vi "Get value by Variant.vi"(8 "error in (no error)":errorcluster, 11 "By-Value Column in":refnum<class "By-Value Column.lvclass">) -> (0 "error out":errorcluster, 2 "Variant":variant, 3 "By-Value Column out":refnum<class "By-Value Column.lvclass">)   [LabVIEW 2020, in "Basic Columns.lvlib" / "By-Value Column.lvclass"]
uses:
  By-Value Column.lvclass
  Column Class/Column Parent.lvclass
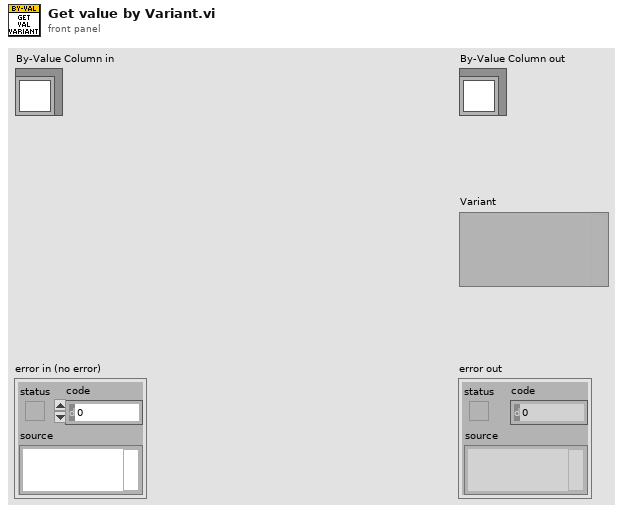
[diagram p1: front panel]
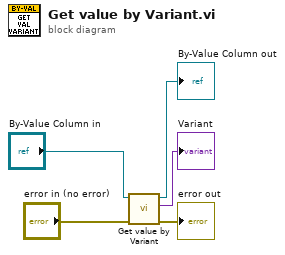
[diagram p0: block diagram]
diagram:
  n1 = call-parent "Get value by Variant.vi"("error in (no error)"="error in (no error)", "Column Parent in"="By-Value Column in") -> ("error out"=→"error out":errorcluster, "Variant"=→"Variant":variant, "Column Parent out"=→"By-Value Column out":refnum<class "By-Value Column.lvclass">)  [unwired: 7 in]
